vi "example_GRecord.vi"() -> ()   [LabVIEW 2020]
uses:
  gclib32.lvlib
panel:
  out "TIME":u16
  in  "IP Address":string="192.168.1.77 --subscribe DR"
  out "Controller ID":string
  out "error out":errorcluster
  in  "stop":bool
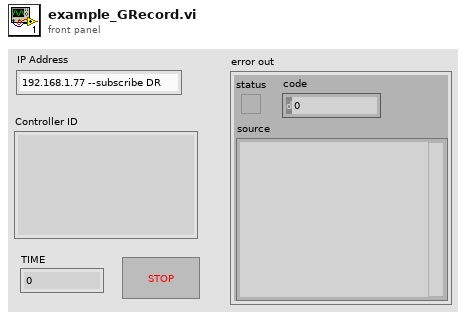
[diagram p1: front panel]
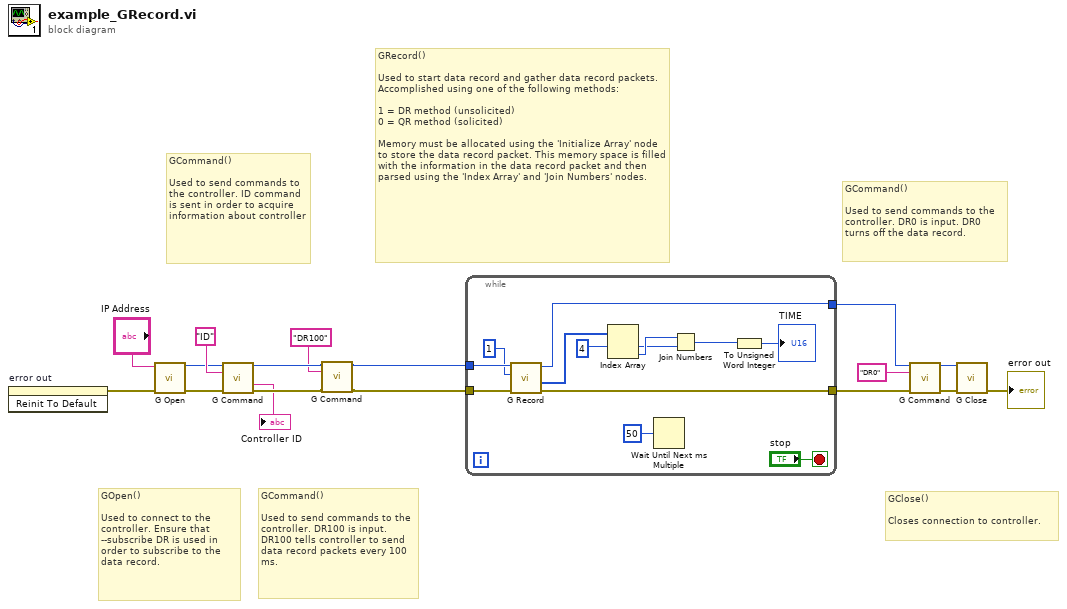
[diagram p0: block diagram]
diagram:
  # "GRecord()\n\nUsed to start data record and gather data record packets. Accomplished using one of the following methods:\n\n1 = DR method (unsolicited)\n0 = QR method (solicited)\n\nMemory must be allocated using the 'Initialize Array' node to store the data record packet. This memory space is filled with the information in the data record packet and then parsed using the 'Index Array' and 'Join Numbers' nodes."
  # "GClose()\n\nCloses connection to controller."
  # "GCommand()\n\nUsed to send commands to the controller. DR0 is input. DR0 turns off the data record."
  # "GCommand()\n\nUsed to send commands to the controller. DR100 is input. DR100 tells controller to send data record packets every 100 ms."
  # "GCommand()\n\nUsed to send commands to the controller. ID command is sent in order to acquire information about controller"
  # "GOpen()\n\nUsed to connect to the controller. Ensure that \n--subscribe DR is used in order to subscribe to the data record."
  n1 = invoke on="error out" class="Clust (strict)" method="Reinit To Default"() -> (error out=w12:errorcluster)  [unwired: 3 in, 2 out]
  n2 = call "G Open.vi"("error in (no error)"=w12, "address"="IP Address") -> ("error out"=w13:errorcluster, "g out"=w14:u32)  [unwired: 7 in]
  n3 = call "G Command.vi"("g"=w14, "command"="ID" ("buffer"), "error in (no error)"=w13) -> ("g out"=w6:u32, "buffer out"=→"Controller ID":string, "error out"=w9:errorcluster)  [unwired: 10 in]
  n4 = call "G Command.vi"("g"=w6, "command"="DR100", "error in (no error)"=w9) -> ("g out"=w7:u32, "error out"=w8:errorcluster)  [unwired: 10 in, 1 out]
  n5 = while {
    tunnel: [w18] -> w1
    tunnel: [w20] -> w3
    tunnel: w7 -> [w23]
    tunnel: w8 -> [w21]
    stop <- "stop" stop-if-true
    n6 = call "G Record.vi"("error in (no error)"=w21, "method"=1, "g"=w23) -> ("error out"=w18:errorcluster, "record out"=w19:u8[], "g out"=w20:u32)  [unwired: 6 in]
    n7 = Index Array "Index Array"(array=w19, index #1=4 ("index")) -> (element #1=w27:u8, element #2=w28:u8)  [unwired: 1 in]
    n8 = Wait Until Next ms Multiple(millisecond multiple=u32 50) -> ()  [unwired: 1 out]
    n9 = Join Numbers(hi=w28, lo=w27) -> ((hi.lo)=w25:u16)
    n10 = To Unsigned Word Integer(number=w25) -> (unsigned 16bit integer=→"TIME":u16)
  }
  n11 = call "G Command.vi"("g"=w3, "command"="DR0", "error in (no error)"=w1) -> ("g out"=w11:u32, "error out"=w10:errorcluster)  [unwired: 10 in, 1 out]
  n12 = call "G Close.vi"("error in (no error)"=w10, "g"=w11) -> ("error out"=→"error out":errorcluster)  [unwired: 9 in]
